vi "SendTCPPackage.vi"(0 "connection ID":refnum<k5>, 1 "command":T1 items=["GarbageCollect", "GetAllObjects", "GetAllObjectsReply", "CleanUp", "G#Event", "RegisterClient", "GetAttributeValue", "GetAttributeValueReply", "GetClassAttributeValue", "GetClassAttributeValueReply", "GetToStringValue", "GetToStringValueReply", "GetClassHierarchy", "GetClassHierarchyReply", "Destroy", "RemoveClient"], 2 "data":string, 4 "timeout ms (200)":i32=200, 5 "error in (no error)":errorcluster, 6 "enabled":bool=TRUE) -> (19 "error out":errorcluster)   [LabVIEW 2017, in "G#DebugServer.lvclass"]
doc: "Sends UPD package."
uses:
  <vilib>/addons/_AddQ/G#DebugServer/G#DebugServer.lvclass
  <vilib>/addons/_AddQ/G#DebugServer/utils/TCPCommand.ctl
  <vilib>/addons/_AddQ/G#Object/G#Object.lvclass
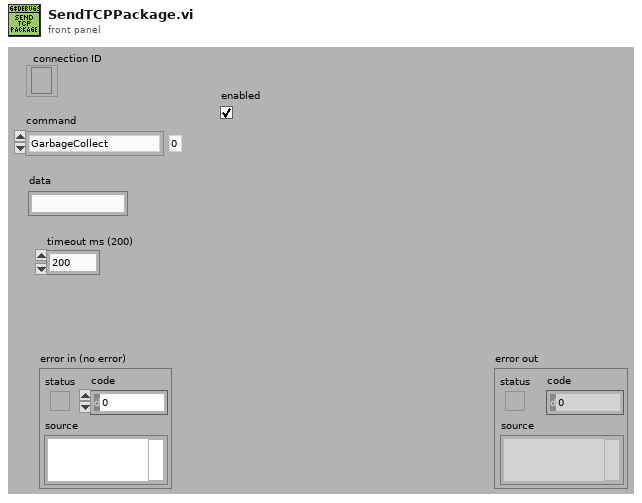
[diagram p1: front panel]
types:
  T1 = typedef "G#DebugServer.lvclass/TCPCommand.ctl" = u8
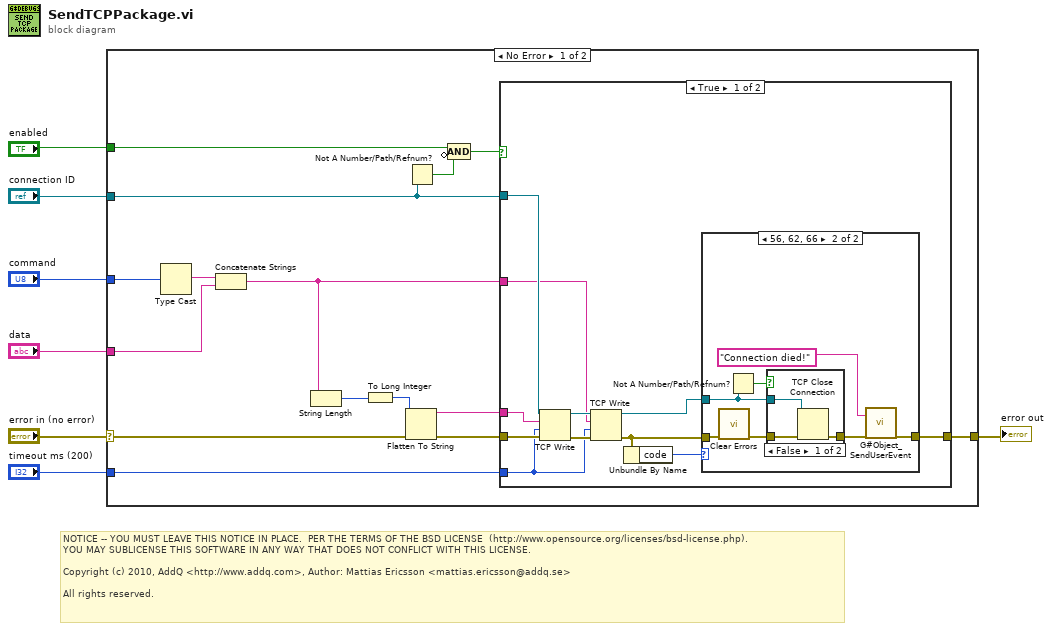
[diagram p0: block diagram]
diagram:
  # "NOTICE -- YOU MUST LEAVE THIS NOTICE IN PLACE.  PER THE TERMS OF THE BSD LICENSE  (http://www.opensource.org/licenses/bsd-license.php).\nYOU MAY SUBLICENSE THIS SOFTWARE IN ANY WAY THAT DOES NOT CONFLICT WITH THIS LICENSE.\n\nCopyright (c) 2010, AddQ <http://www.addq.com>, Author: Mattias Ericsson <mattias.ericsson@addq.se>\n\nAll rights reserved."
  n1 = case shown="No Error" "error in (no error)" {
    selector: "error in (no error)" -> [w15 w47]
    tunnel: [w22 w47] -> w6
    tunnel: "command" -> [w21 _]
    tunnel: "data" -> [w18 _]
    tunnel: "connection ID" -> [w19 _]
    tunnel: "timeout ms (200)" -> [w11 _]
    tunnel: "enabled" -> [w9 _]
    frame No Error {
      n2 = Type Cast(x=w21) -> (*(type *) &x=w20:string)  [unwired: 1 in]
      n3 = Concatenate Strings(w20, w18) -> (w17:string)
      n4 = String Length(string=w17) -> (length=w16:i32)
      n5 = To Long Integer(number=w16) -> (32bit integer=w13:i32)
      n6 = Flatten To String(anything=w13, error in (no error)=w15) -> (data string=w12:string, error out=w14:errorcluster)  [unwired: 2 in, 1 out]
      n7 = Not A Number/Path/Refnum?(number/path/refnum=w19) -> (NaN/Path/Refnum?=w10:bool)
      n8 = Compound Arithmetic op=AND(w9, invert w10) -> (w8:bool)
      n9 = case shown="True" w8 {
        tunnel: w14 -> [w33 w46]
        tunnel: [w24 w46] -> w22
        tunnel: w19 -> [w30 _]
        tunnel: w17 -> [w28 _]
        tunnel: w12 -> [w29 _]
        tunnel: w11 -> [w27 _]
        frame True {
          n10 = TCP Write(connection ID=w30, data in=w29, error in (no error)=w33, 9:w27) -> (connection ID out=w31:refnum<k5>, error out=w32:errorcluster)  [unwired: 1 out]
          n11 = TCP Write(connection ID=w31, data in=w28, error in (no error)=w32, 9:w27) -> (connection ID out=w23:refnum<k5>, error out=w26:errorcluster)  [unwired: 1 out]
          n12 = Unbundle By Name(w26) -> ("code"=w25:i32)
          n13 = case shown="56, 62, 66" w25 {
            tunnel: w26 -> [w34 w41]
            tunnel: [w34 w39] -> w24
            tunnel: w23 -> [_ w36]
            frame 0, Default {
            }
            frame 56, 62, 66 {
              n14 = call <vilib>:"Clear Errors.vi"("error in (no error)"=w41) -> ("error out"=w40:errorcluster)  [unwired: 5 in, 1 out]
              n15 = Not A Number/Path/Refnum?(number/path/refnum=w36) -> (NaN/Path/Refnum?=w35:bool)
              n16 = case shown="False" w35 {
                tunnel: w40 -> [w44 w45]
                tunnel: [w43 w45] -> w38
                tunnel: w36 -> [w42 _]
                frame False {
                  n17 = TCP Close Connection(connection ID=w42, error in (no error)=w44) -> (error out=w43:errorcluster)  [unwired: 1 in, 1 out]
                }
                frame True {
                }
              }
              n18 = call <vilib>:"G#Object_SendUserEvent.vi"("text"="Connection died!", "error in (no error)"=w38) -> ("error out"=w39:errorcluster)  [unwired: 16 in, 1 out]
            }
          }
        }
        frame False {
          # "Don't send anything!"
        }
      }
    }
    frame Error {
    }
  }
  "error out" <- w6
